vi "Bezier Curve sub-part.vi"(8 "Q":cluster{cdb, cdb}[](array[cluster]), 9 "degree":i32, 10 "Fourier Matrix":cdb[](array[numeric]), 11 "position":dbl) -> (2 "y arr":dbl[](array[numeric]), 3 "x arr":dbl[](array[numeric]))   [LabVIEW 2025]
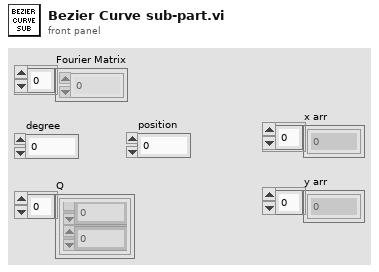
[diagram p1: front panel]
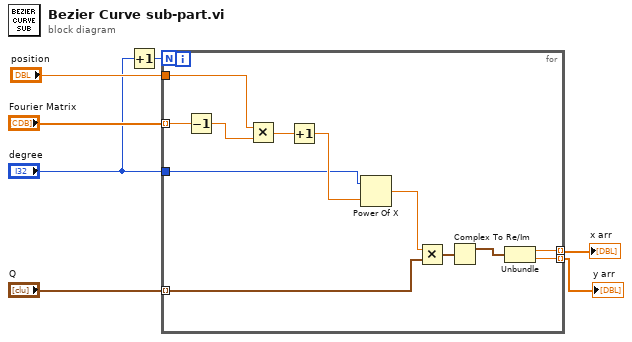
[diagram p0: block diagram]
diagram:
  n1 = Increment(x="degree") -> (x+1=w2:i32)
  n2 = for {
    N: w2 -> [_]
    tunnel: "Q" -> [w12] mode=indexing
    tunnel: "degree" -> [w13]
    tunnel: "position" -> [w8]
    tunnel: [w17] -> w5 mode=indexing
    tunnel: [w16] -> w6 mode=indexing
    tunnel: "Fourier Matrix" -> [w15] mode=indexing
    n3 = Decrement(x=w15) -> (x-1=w14:cdb)
    n4 = Multiply(x=w8, y=w14) -> (x*y=w19:cdb)
    n5 = Increment(x=w19) -> (x+1=w18:cdb)
    n6 = Power Of X(1:w18, 2:w13) -> (0:w11:cdb)
    n7 = Multiply(x=w11, y=w12) -> (x*y=w10:cluster{cdb, cdb})
    n8 = Complex To Re/Im(x + iy=w10) -> (x=w9:cluster{dbl, dbl})  [unwired: 1 out]
    n9 = Unbundle(w9) -> (w17:dbl, w16:dbl)
  }
  "y arr" <- w6
  "x arr" <- w5
